vi "Part 1.vi"(11 "Input":string) -> (3 "Output":i64)   [LabVIEW 2021]
uses:
  1bddd3f3-30de-4f3d-a608-9edb45d621d8.vi
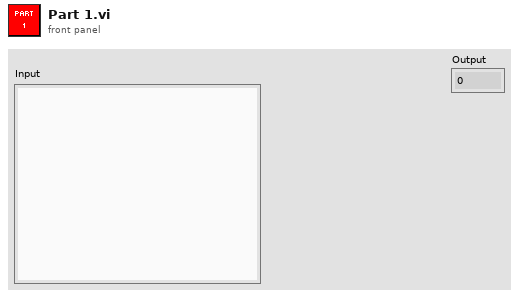
[diagram p1: front panel]
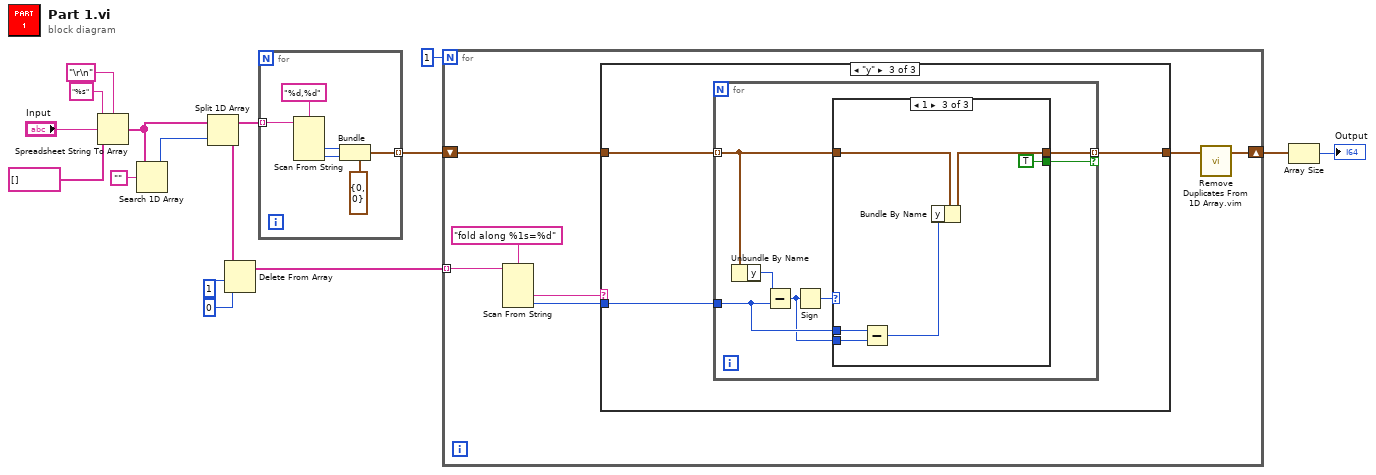
[diagram p0: block diagram]
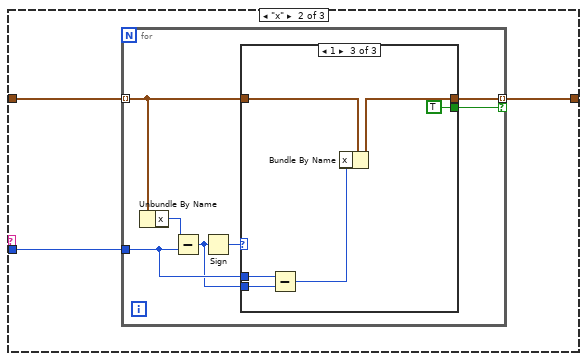
[diagram p3: hidden frame]
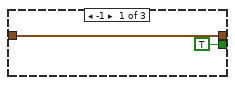
[diagram p4: hidden frame]
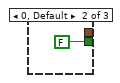
[diagram p5: hidden frame]
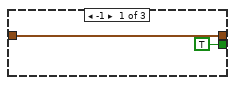
[diagram p6: hidden frame]
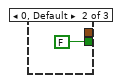
[diagram p7: hidden frame]
diagram:
  n1 = Spreadsheet String To Array(delimiter (Tab)="\r\n", format string="%s", spreadsheet string="Input", array type (2D Dbl)=string[] []) -> (array=w11:string[])
  n2 = Search 1D Array(1D array=w11, element="") -> (index of element=w10:i32)  [unwired: 1 in]
  n3 = Split 1D Array(array=w11, index=w10) -> (first subarray=w5:string[], second subarray=w6:string[])
  n4 = Delete From Array(array=w6, length=1 ("index"), index=0) -> (array with subset deleted=w7:string[])  [unwired: 1 out]
  n5 = for {
    tunnel: w5 -> [w22] mode=indexing
    tunnel: [w19] -> w4 mode=indexing
    n6 = Scan From String(format string="%d,%d", input string=w22) -> (output 1=w20:i32, output 2=w18:i32)  [unwired: 4 in, 3 out]
    n7 = Bundle(cluster=cluster{"x":i32, "y":i32} {"x"=0, "y"=0}, "x"=w20, "y"=w18) -> (w19:cluster{"x":i32, "y":i32})
  }
  n8 = for {
    N: 1 -> [_]
    tunnel: w7 -> [w29] mode=indexing
    shift-right: [w23] -> w1
    shift-left: w4 -> [w25]
    n9 = Scan From String(format string="fold along %1s=%d", input string=w29) -> (output 1=w27:string, output 2=w26:i32)  [unwired: 4 in, 3 out]
    n10 = case shown="\"y\"" w27 {
      tunnel: w26 -> [_ w33 w52]
      tunnel: w25 -> [w30 w32 w51]
      tunnel: [w30 w31 w50] -> w24
      frame Default {
      }
      frame "x" {
        n11 = for {
          tunnel: w32 -> [w38] mode=indexing
          tunnel: w33 -> [w35]
          tunnel: [w37] -> w31 mode=indexing if=w36
          n12 = Unbundle By Name(w38) -> ("x"=w39:i32)
          n13 = Subtract(x=w39, y=w35) -> (x-y=w34:i32)
          n14 = Sign(1:w34) -> (0:w40:i32)
          n15 = case shown="1" w40 {
            tunnel: [w42 _ w47] -> w37
            tunnel: w38 -> [w42 _ w48]
            tunnel: [TRUE FALSE TRUE] -> w36
            tunnel: w35 -> [_ _ w46]
            tunnel: w34 -> [_ _ w45]
            frame -1 {
            }
            frame 0, Default {
            }
            frame 1 {
              n16 = Subtract(x=w46, y=w45) -> (x-y=w44:i32)
              n17 = Bundle By Name(cluster=w48, "x"=w44) -> (w47:cluster{"x":i32, "y":i32})
            }
          }
        }
      }
      frame "y" {
        n18 = for {
          tunnel: w51 -> [w57] mode=indexing
          tunnel: w52 -> [w54]
          tunnel: [w56] -> w50 mode=indexing if=w55
          n19 = Unbundle By Name(w57) -> ("y"=w58:i32)
          n20 = Subtract(x=w58, y=w54) -> (x-y=w53:i32)
          n21 = Sign(1:w53) -> (0:w59:i32)
          n22 = case shown="1" w59 {
            tunnel: [w61 _ w66] -> w56
            tunnel: w57 -> [w61 _ w67]
            tunnel: [TRUE FALSE TRUE] -> w55
            tunnel: w54 -> [_ _ w65]
            tunnel: w53 -> [_ _ w64]
            frame -1 {
            }
            frame 0, Default {
            }
            frame 1 {
              n23 = Subtract(x=w65, y=w64) -> (x-y=w63:i32)
              n24 = Bundle By Name(cluster=w67, "y"=w63) -> (w66:cluster{"x":i32, "y":i32})
            }
          }
        }
      }
    }
    n25 = call "Remove Duplicates From 1D Array.vim"("array"=w24) -> ("array with duplicates removed"=w23:cluster{"x":i32, "y":i32}[])  [unwired: 10 in]
  }
  n26 = Array Size(array=w1) -> (size(s)=→"Output":i32)
